vi "Turret_Main_Calc.vi"(8 "At Maximum Angle":bool, 9 "At Minimum Angle":bool, 10 "Desired Horizontal Offset":dbl, 11 "Current Horizontal Position":dbl) -> (2 "Target In Deadzone":bool, 3 "Output Turret Position":dbl)   [LabVIEW 2012]
panel:
  out "error out":errorcluster
  in  "Position Resolution":dbl=0.01
  in  "Minimum Angle":dbl
  # "Encoder Units"
  # "Encoder Units"
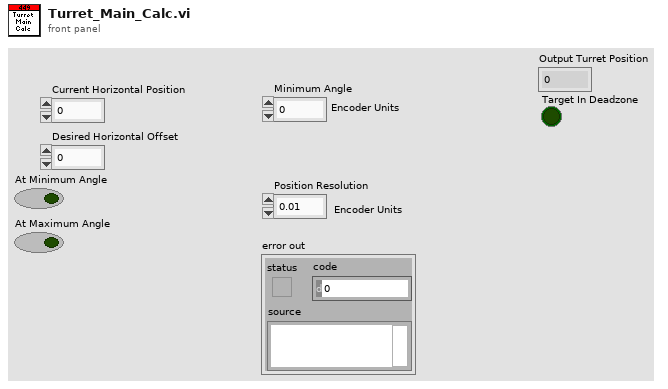
[diagram p1: front panel]
types:
  T1 = typedef "WPI_MotorControlDeviceRef.ctl" = cluster{"DeviceStatus":errorcluster, "Type":enum16{"PWM", "CAN"}, "PWM":cluster{"Digital Module":T2, "PWM Channel":T3, "DeadBand":T4}, "CAN":cluster{"Device Number":u8, "Control Mode":T5, "Semaphore":T6, "Max Vout":dbl}, "Invert":bool, "TransformRef":T7, "InvTransformRef":T7}
  T2 = typedef "FPGA_TypedefDigitalModule.ctl" = enum16{"Digital Module 1", "Digital Module 2"}
  T3 = typedef "FPGA_DIOPWMChannel.ctl" = enum8{"PWM 1", "PWM 2", "PWM 3", "PWM 4", "PWM 5", "PWM 6", "PWM 7", "PWM 8", "PWM 9", "PWM 10", "Invalid"}
  T4 = typedef "WPI_PWMDeadband.ctl" = cluster{"Name":string, "maxPositivePwm":i32, "minPositivePwm":i32, "centerPwm":i32, "maxNegativePwm":i32, "minNegativePwm":i32, "angularRange":u16}
  T5 = typedef "WPI_CANJaguar_ControlMode.ctl" = enum8{"Percent VBus", "Current", "Speed", "Position", "Voltage"}
  T6 = typedef "Semaphore RefNum" = refnum<k1>
  T7 = typedef "WPI_PWMTransform_ConPane.ctl" = refnum<vi>
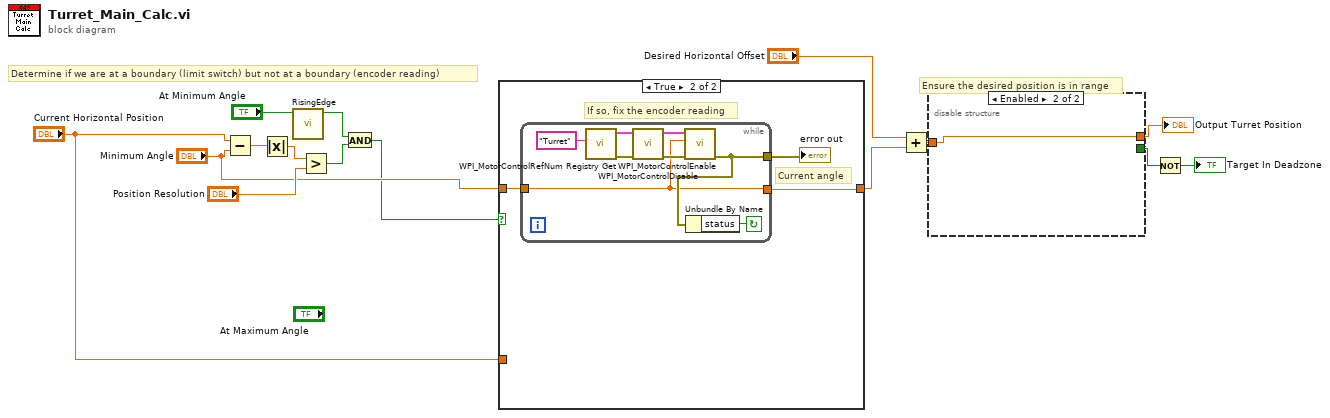
[diagram p0: block diagram]
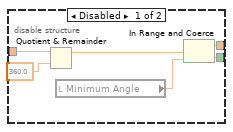
[diagram p2: hidden frame]
diagram:
  # "Determine if we are at a boundary (limit switch) but not at a boundary (encoder reading)"
  # "Ensure the desired position is in range"
  n1 = Subtract(x="Current Horizontal Position", y="Minimum Angle") -> (x-y=w14:dbl)
  n2 = Absolute Value(x=w14) -> (abs(x)=w13:dbl)
  n3 = call "RisingEdge.vi"("BooleanIn"="At Minimum Angle") -> ("BooleanOut"=w1:bool)  [unwired: 10 in]
  n4 = Greater?(x=w13, y="Position Resolution") -> (0:w12:bool)
  n5 = And(x=w1, y=w12) -> (x .and. y?=w2:bool)
  n6 = case shown="True" w2 {
    tunnel: "Minimum Angle" -> [_ w19]
    tunnel: [w16 w17] -> w9
    tunnel: "Current Horizontal Position" -> [w16 _]
    frame False {
      # "No problem with the encoder reading; keep going"
      # "Current angle"
    }
    frame True {
      # "Current angle"
      # "If so, fix the encoder reading"
      n7 = while {
        tunnel: w19 -> [w20]
        tunnel: [w22] -> w18
        tunnel: [w20] -> w17
        stop <- w21 continue-if-true
        n8 = call <vilib>:"WPI_MotorControlRefNum Registry Get.vi"("refnum name"="Turret") -> ("error out"=w26:errorcluster, "MotorControlDevRef"=w25:T1)  [unwired: 9 in]
        n9 = call <vilib>:"WPI_MotorControlDisable.vi"("error in (no error)"=w26, "MotorControlDevRef"=w25) -> ("error out"=w24:errorcluster, "MotorControlDevRef"=w23:T1)  [unwired: 8 in]
        n10 = call <vilib>:"WPI_MotorControlEnable.vi"("error in (no error)"=w24, "Encoder Initial Position"=w20, "CAN Jaguar Ref"=w23) -> ("error out"=w22:errorcluster)  [unwired: 7 in, 1 out]
        n11 = Unbundle By Name(w22) -> ("status"=w21:bool)
      }
      "error out" <- w18
    }
  }
  n12 = Add(x="Desired Horizontal Offset", y=w9) -> (x+y=w7:dbl)
  n13 = disable-structure shown="Enabled" {
    disable-tunnel: w7 -> [w32 w34]
    disable-tunnel: [w29 w34] -> w6
    disable-tunnel: [w28 _] -> w5
    frame Disabled {
      n14 = Quotient & Remainder(x=w32, y=360.0) -> (x-y*floor(x/y)=w30:dbl)  [unwired: 1 out]
      n15 = local read "Minimum Angle"() -> (w33:dbl)
      n16 = In Range and Coerce(x=w30, lower limit=w33) -> (coerced(x)=w29:dbl, In Range?=w28:bool)  [unwired: 1 in]
    }
    frame Enabled {
    }
  }
  "Output Turret Position" <- w6
  n17 = Not(x=w5) -> (.not. x?=→"Target In Deadzone":bool)
